vi "fp button handler_MD.vi"(5 "dummy error input (just for timing purposes)":errorcluster) -> ()   [LabVIEW 2012]
uses:
  <vilib>/Utility/VariantDataType/Type.ctl
  GFG/GFGallGet.vi
  GFG/GFGfpRefGet.vi
  GFG/GFG library.lvlib
  <vilib>/Utility/VariantDataType/VariantType.lvlib
panel:
  out "Source VI":string
  in  "stop":bool
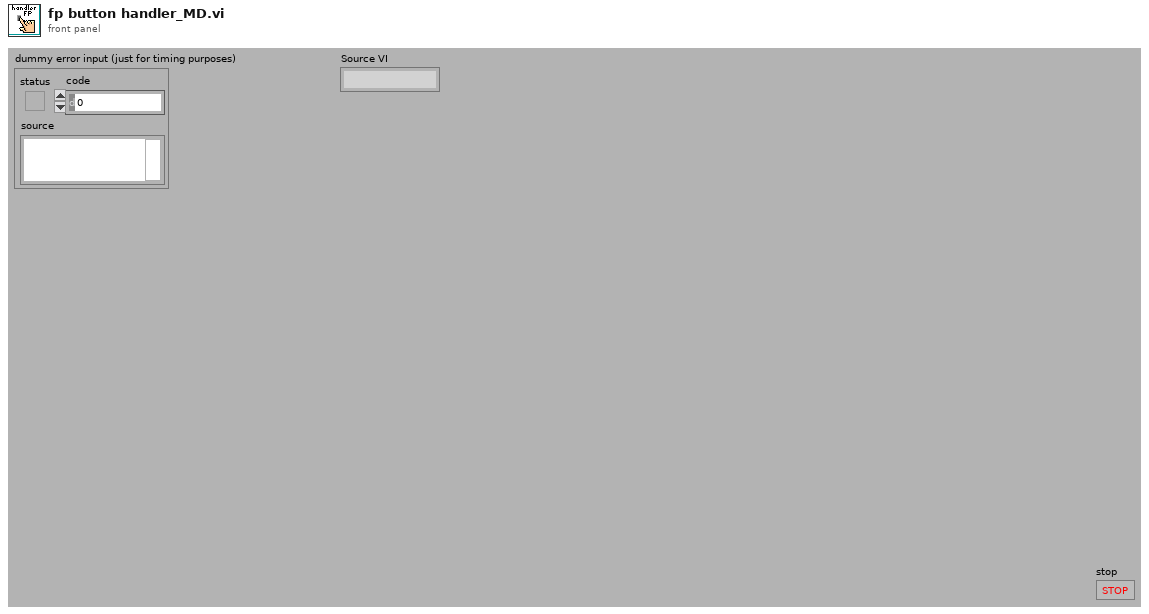
[diagram p1: front panel]
types:
  T1 = typedef "VariantType.lvlib/Type.ctl" = enum8{"Invalid Type", "Void", "I8", "I16", "I32", "I64", "U8", "U16", "U32", "U64", "Single Float", "Double Float", "Extended Float", "Single Complex", "Double Complex", "Extended Complex", "Enum U8", "Enum U16", "Enum U32", "Enum U64", "Single Float With Unit", "Double Float With Unit", "Extended Float With Unit", "Single Complex with Unit", "Double Complex with Unit", "Extended Complex with Unit", "Boolean", "String", "Path", "Picture", "Tag", "Array", "Cluster", "Variant", "LV Variant", "Waveform", "Timestamp", "Digital Waveform", "Digital Data", "ExpressData", "Refnum", "External Data", "VI", "Poly VI", "LabVIEW Class Instance", "Fixed Point"}
  T2 = cluster{"Variable Name Out":string, "Data Type Out":T1, "Variant Out":variant}[]
  T3 = cluster{"WaveformChartRef":refnum<vi>, "DigitalRef":refnum<vi>, "ArrayRef":refnum<vi>, "TabControlRef":refnum<vi>, "EnumRef":refnum<vi>, "RingRef":refnum<vi>, "BooleanRef":refnum<vi>, "KnobRef":refnum<vi>, "SlideRef":refnum<vi>, "PathRef":refnum<vi>, "StringRef":refnum<vi>, "ComboBox":refnum<vi>, "WaveformGraphRef":refnum<vi>}
  T4 = enum8{"Enabled", "Disabled", "Disabled and Grayed Out"}
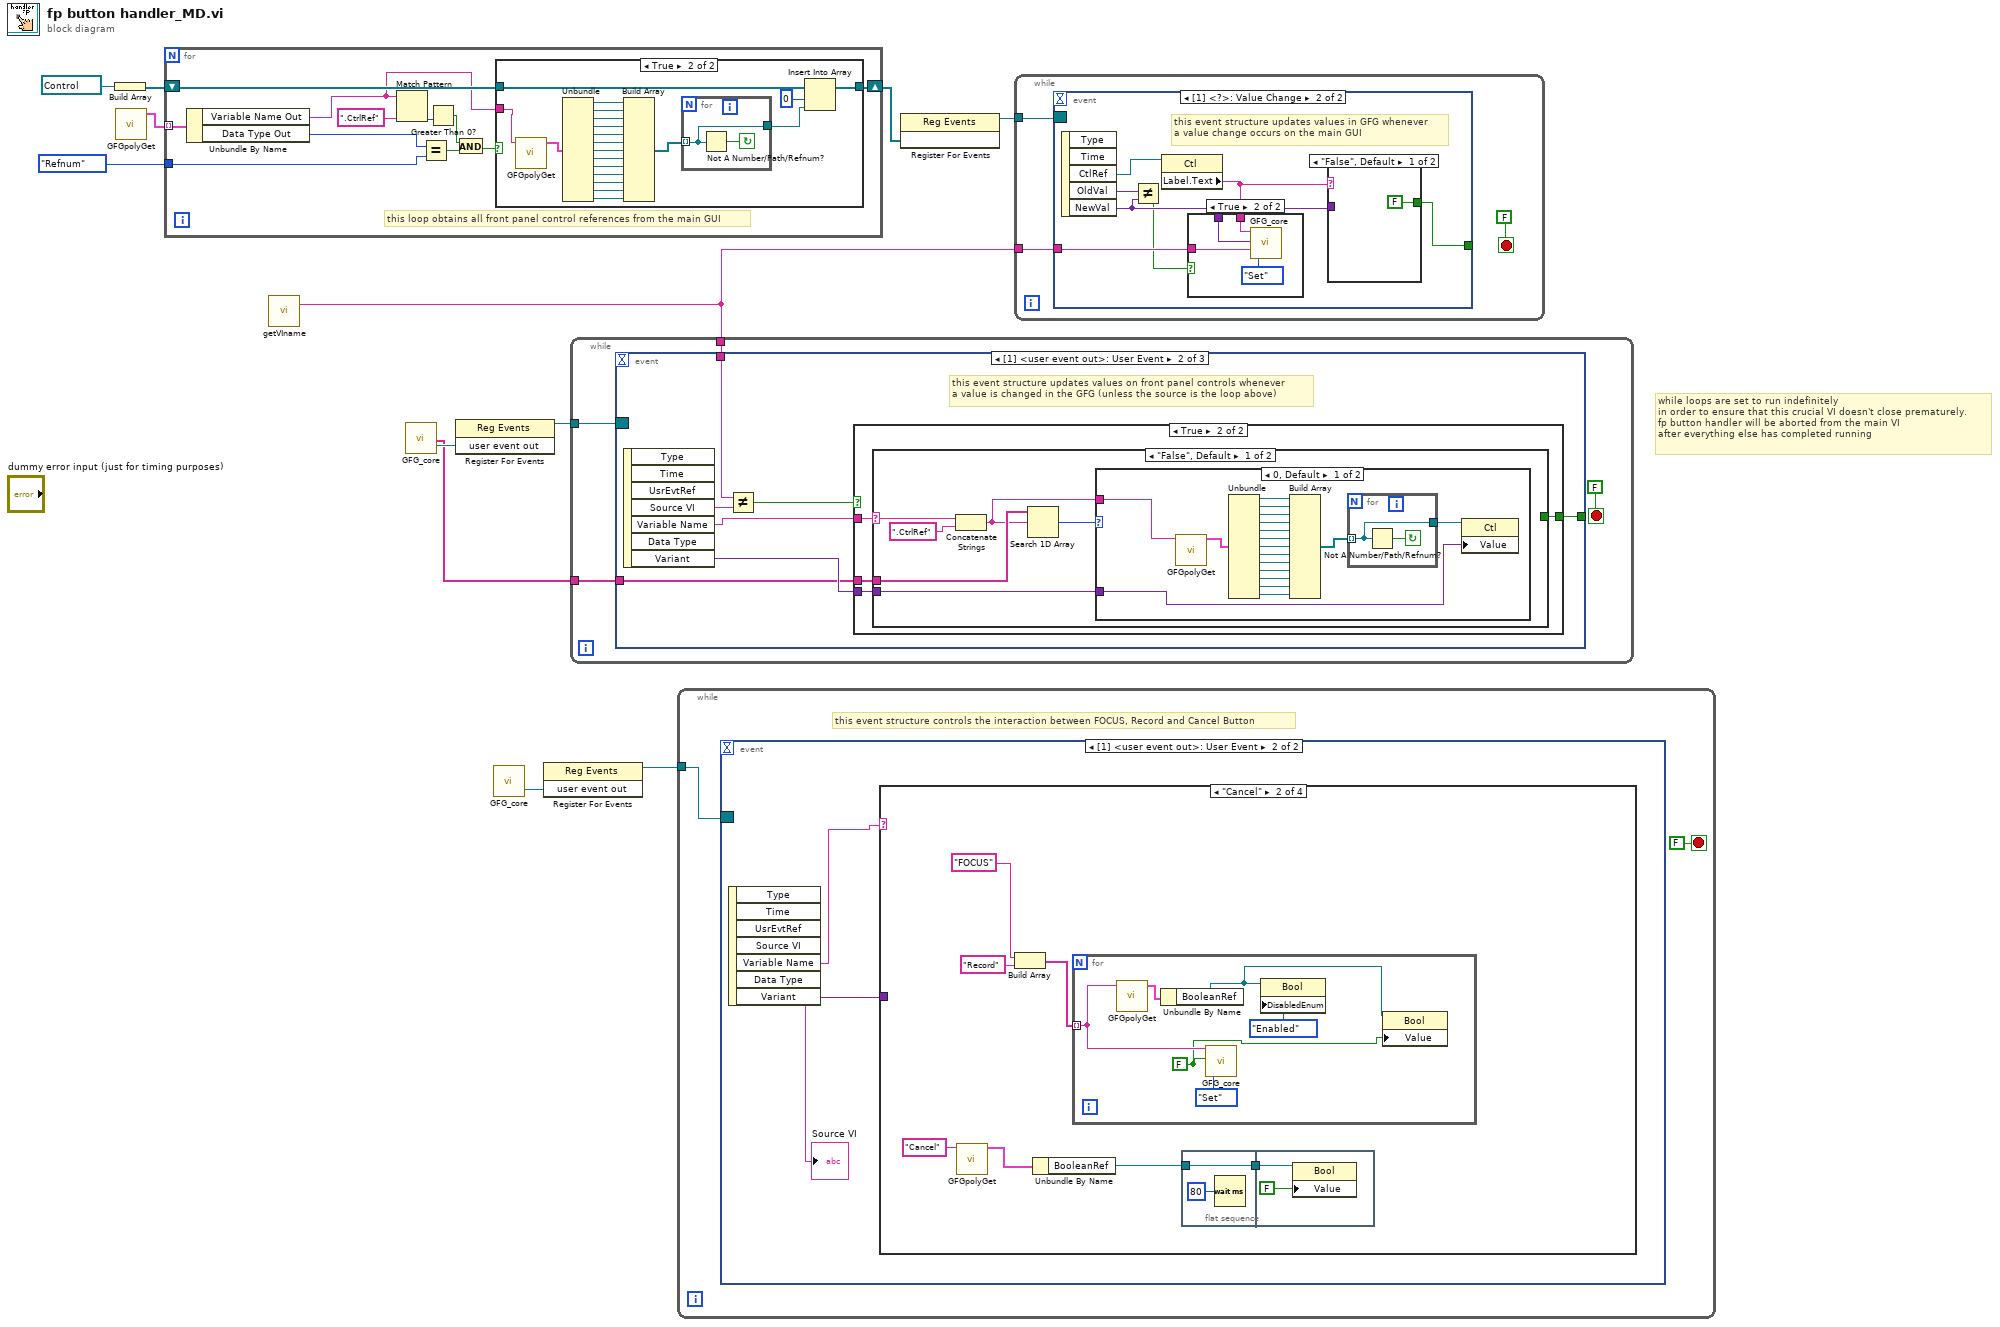
[diagram p0: block diagram]
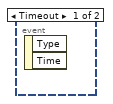
[diagram p2: hidden frame]
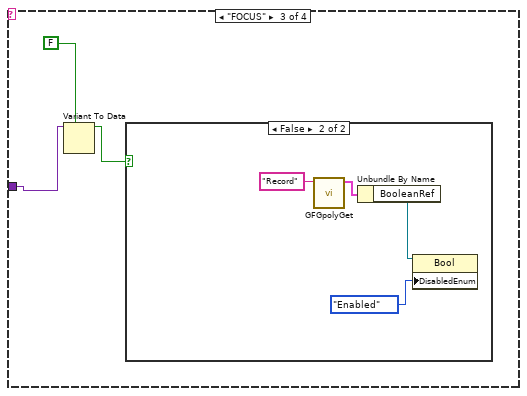
[diagram p4: hidden frame]
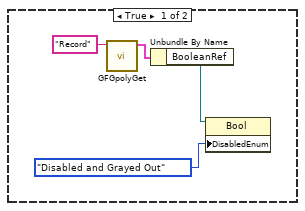
[diagram p5: hidden frame]
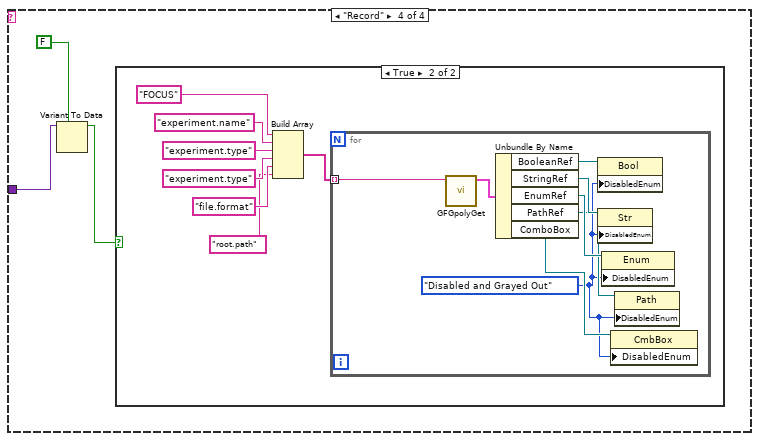
[diagram p6: hidden frame]
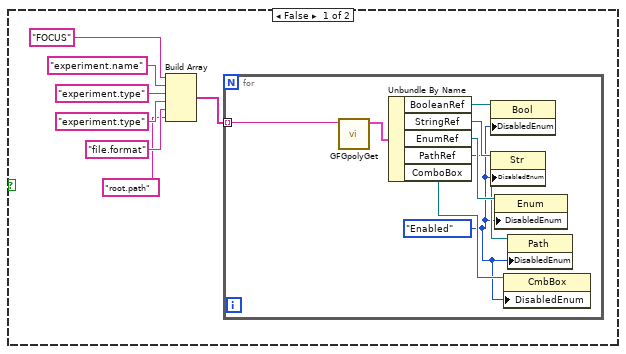
[diagram p7: hidden frame]
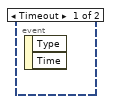
[diagram p8: hidden frame]
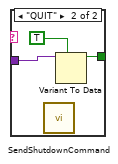
[diagram p10: hidden frame]
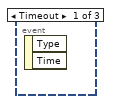
[diagram p12: hidden frame]
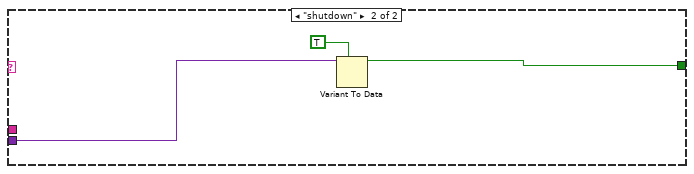
[diagram p15: hidden frame]
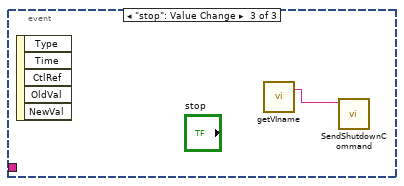
[diagram p16: hidden frame]
diagram:
  # "while loops are set to run indefinitely\nin order to ensure that this crucial VI doesn't close prematurely.\nfp button handler will be aborted from the main VI \nafter everything else has completed running"
  n1 = Build Array(refnum<vi> refnum ("DigitalRef")) -> (w6:refnum<vi>[])
  n2 = call-poly "GFGpolyGet.vi"() -> ("Array of Clusters of Variables"=w9:T2)  [unwired: 10 in, 1 out]
  n3 = for {
    tunnel: w9 -> [w23] mode=indexing
    tunnel: Type."Refnum" ("Data Type Out") -> [w21]
    shift-right: [w19] -> w5
    shift-left: w6 -> [w20]
    # "this loop obtains all front panel control references from the main GUI"
    n4 = Unbundle By Name(w23) -> ("Variable Name Out"=w13:string, "Data Type Out"=w22:T1)
    n5 = Match Pattern(string=w13, regular expression=".CtrlRef" ("string")) -> (offset past match=w17:i32)  [unwired: 1 in, 3 out]
    n6 = Equal?(x=w22, y=w21) -> (x = y?=w14:bool)
    n7 = Greater Than 0?(x=w17) -> (x > 0?=w15:bool)
    n8 = And(x=w15, y=w14) -> (x .and. y?=w16:bool)
    n9 = case shown="True" w16 {
      tunnel: w20 -> [w24 w30]
      tunnel: [w24 w29] -> w19
      tunnel: w13 -> [_ w27]
      frame False {
      }
      frame True {
        n10 = call-poly "GFGpolyGet.vi"("Variable Name in"=w27) -> ("output cluster"=w32:T3)  [unwired: 9 in, 1 out]
        n11 = Unbundle(w32) -> ("WaveformChartRef"=w33:refnum<vi>, "DigitalRef"=w34:refnum<vi>, "ArrayRef"=w35:refnum<vi>, "TabControlRef"=w36:refnum<vi>, "EnumRef"=w37:refnum<vi>, "RingRef"=w38:refnum<vi>, "BooleanRef"=w39:refnum<vi>, "KnobRef"=w40:refnum<vi>, "SlideRef"=w41:refnum<vi>, "PathRef"=w42:refnum<vi>, "StringRef"=w43:refnum<vi>, "ComboBox"=w26:refnum<vi>, "WaveformGraphRef"=w25:refnum<vi>)
        n12 = Build Array(w33, w34, w35, w36, w37, w38, w39, w40, w41, w42, w43, w26, w25) -> (w44:refnum<vi>[])
        n13 = for {
          tunnel: w44 -> [w45] mode=indexing
          tunnel: [w45] -> w31
          stop <- w46 continue-if-true
          n14 = Not A Number/Path/Refnum?(number/path/refnum=w45) -> (NaN/Path/Refnum?=w46:bool)
        }
        n15 = Insert Into Array(array=w30, index=0, new element=w31) -> (w29:refnum<vi>[])
      }
    }
  }
  n16 = call "getVIname.vi"() -> ("VI name"=w1:string)  [unwired: 19 in]
  n17 = call "GFG_core.vi"() -> ("All Variable Names Out"=w10:string[], "user event out"=w11:refnum<user-event>)  [unwired: 13 in, 5 out]
  n18 = register-events(w11) -> (reference out=w12:refnum<event-registration>)  [unwired: 2 in, 1 out]
  n19 = call "GFG_core.vi"() -> ("user event out"=w3:refnum<user-event>)  [unwired: 13 in, 6 out]
  n20 = register-events(w3) -> (reference out=w2:refnum<event-registration>)  [unwired: 2 in, 1 out]
  n21 = while {
    tunnel: w12 -> [w50]
    tunnel: w10 -> [w49]
    tunnel: w1 -> [w48]
    stop <- FALSE stop-if-true
    n22 = event shown="[1] <user event out>: User Event" {
      selector: w50 -> [_ _ _]
      dyn-events: _ -> [_ _ _]
      timeout: _ -> [_ _ _]
      tunnel: [_ w55 _] -> _
      tunnel: w49 -> [_ w54 _]
      tunnel: w48 -> [_ w53 _]
      event Timeout {
        n23 = event-data() -> ()  [unwired: 1 in, 2 out]
      }
      event User Event {
        # "this event structure updates values on front panel controls whenever\na value is changed in the GFG (unless the source is the loop above)"
        n24 = event-data() -> ("Source VI"=w52:string, "Variable Name"=w57:string, "Variant"=w56:variant)  [unwired: 1 in, 4 out]
        n25 = Not Equal?(x=w53, y=w52) -> (x != y?=w51:bool)
        n26 = case shown="True" w51 {
          tunnel: w57 -> [_ w61]
          tunnel: w56 -> [_ w60]
          tunnel: [_ w59] -> w55
          tunnel: w54 -> [_ w58]
          frame False {
          }
          frame True {
            n27 = case shown="\"False\", Default" w61 {
              selector: w61 -> [w66 _]
              tunnel: w60 -> [w62 w90]
              tunnel: [_ w88] -> w59
              tunnel: w58 -> [w65 _]
              frame "False", Default {
                n28 = Concatenate Strings(w66, ".CtrlRef" ("string")) -> (w63:string)
                n29 = Search 1D Array(1D array=w65, element=w63) -> (index of element=w64:i32)  [unwired: 1 in]
                n30 = case shown="0, Default" w64 {
                  tunnel: w63 -> [w85 _]
                  tunnel: w62 -> [w70 _]
                  frame 0, Default {
                    n31 = call-poly "GFGpolyGet.vi"("Variable Name in"=w85) -> ("output cluster"=w84:T3)  [unwired: 9 in, 1 out]
                    n32 = Unbundle(w84) -> ("WaveformChartRef"=w83:refnum<vi>, "DigitalRef"=w82:refnum<vi>, "ArrayRef"=w81:refnum<vi>, "TabControlRef"=w80:refnum<vi>, "EnumRef"=w79:refnum<vi>, "RingRef"=w78:refnum<vi>, "BooleanRef"=w77:refnum<vi>, "KnobRef"=w76:refnum<vi>, "SlideRef"=w75:refnum<vi>, "PathRef"=w74:refnum<vi>, "StringRef"=w73:refnum<vi>, "ComboBox"=w69:refnum<vi>, "WaveformGraphRef"=w68:refnum<vi>)
                    n33 = Build Array(w83, w82, w81, w80, w79, w78, w77, w76, w75, w74, w73, w69, w68) -> (w72:refnum<vi>[])
                    n34 = for {
                      tunnel: w72 -> [w86] mode=indexing
                      tunnel: [w86] -> w71
                      stop <- w87 continue-if-true
                      n35 = Not A Number/Path/Refnum?(number/path/refnum=w86) -> (NaN/Path/Refnum?=w87:bool)
                    }
                    n36 = property class="Ctl"(reference=w71, "Value"=w70) -> ()  [unwired: 1 in, 2 out]
                  }
                  frame -1 {
                  }
                }
              }
              frame "shutdown" {
                n37 = Variant To Data(type=TRUE ("want seconds? (F)"), Variant=w90) -> (data=w88:bool)  [unwired: 1 in, 1 out]
              }
            }
          }
        }
      }
      event "stop": Value Change {
        n38 = event-data() -> ()  [unwired: 1 in, 5 out]
        n39 = call "getVIname.vi"() -> ("VI name"=w91:string)  [unwired: 19 in]
        n40 = call "SendShutdownCommand.vi"("Source VI"=w91) -> ()  [unwired: 11 in]
      }
    }
  }
  n41 = while {
    tunnel: w2 -> [w93]
    stop <- FALSE stop-if-true
    # "this event structure controls the interaction between FOCUS, Record and Cancel Button"
    n42 = event shown="[1] <user event out>: User Event" {
      selector: w93 -> [_ _]
      dyn-events: _ -> [_ _]
      timeout: _ -> [_ _]
      event Timeout {
        n43 = event-data() -> ()  [unwired: 1 in, 2 out]
      }
      event User Event {
        n44 = event-data() -> ("Source VI"=→"Source VI":string, "Variable Name"=w96:string, "Variant"=w95:variant)  [unwired: 1 in, 4 out]
        n45 = case shown="\"Cancel\"" w96 {
          tunnel: w95 -> [_ _ w115 w127]
          frame "False", Default {
          }
          frame "Cancel" {
            n46 = call-poly "GFGpolyGet.vi"("Variable Name in"="Cancel") -> ("output cluster"=w99:T3)  [unwired: 9 in, 1 out]
            n47 = Build Array("FOCUS" ("Variable Name in"), "Record" ("element")) -> (w101:string[])
            n48 = Unbundle By Name(w99) -> ("BooleanRef"=w98:refnum<vi>)
            n49 = for {
              tunnel: w101 -> [w110] mode=indexing
              w108 = FALSE
              n50 = call-poly "GFGpolyGet.vi"("Variable Name in"=w110) -> ("output cluster"=w112:T3)  [unwired: 9 in, 1 out]
              n51 = Unbundle By Name(w112) -> ("BooleanRef"=w109:refnum<vi>)
              n52 = call "GFG_core.vi"("Variable Name in"=w110, "Variant in"=w108, "Action"=enum16{"Init", "Set", "Get"}."Set") -> ()  [unwired: 10 in, 7 out]
              n53 = property class="Bool"(reference=w109, "DisabledEnum"=T4."Enabled" ("Disabled")) -> ()  [unwired: 1 in, 2 out]
              n54 = property class="Bool"(reference=w109, "Value"=w108) -> ()  [unwired: 1 in, 2 out]
            }
            n55 = flat-sequence {
              tunnel: w98 -> [w105]
              tunnel: [w105] -> w97
              tunnel: w97 -> [w107]
              frame #0 {
                n56 = Wait (ms)(milliseconds to wait=u32 80) -> ()  [unwired: 1 out]
              }
              frame #1 {
                n57 = property class="Bool"(reference=w107, "Value"=FALSE) -> ()  [unwired: 1 in, 2 out]
              }
            }
          }
          frame "FOCUS" {
            n58 = Variant To Data(type=FALSE ("NewVal"), Variant=w115) -> (data=w114:bool)  [unwired: 1 in, 1 out]
            n59 = case shown="False" w114 {
              frame True {
                n60 = call-poly "GFGpolyGet.vi"("Variable Name in"="Record") -> ("output cluster"=w118:T3)  [unwired: 9 in, 1 out]
                n61 = Unbundle By Name(w118) -> ("BooleanRef"=w117:refnum<vi>)
                n62 = property class="Bool"(reference=w117, "DisabledEnum"=T4."Disabled and Grayed Out" ("Disabled")) -> ()  [unwired: 1 in, 2 out]
              }
              frame False {
                n63 = call-poly "GFGpolyGet.vi"("Variable Name in"="Record") -> ("output cluster"=w122:T3)  [unwired: 9 in, 1 out]
                n64 = Unbundle By Name(w122) -> ("BooleanRef"=w121:refnum<vi>)
                n65 = property class="Bool"(reference=w121, "DisabledEnum"=T4."Enabled" ("Disabled")) -> ()  [unwired: 1 in, 2 out]
              }
            }
          }
          frame "Record" {
            n66 = Variant To Data(type=FALSE ("NewVal"), Variant=w127) -> (data=w125:bool)  [unwired: 1 in, 1 out]
            n67 = case shown="True" w125 {
              frame False {
                n68 = Build Array("FOCUS" ("Variable Name in"), "experiment.name" ("element"), "experiment.type" ("element"), "experiment.type" ("element"), "file.format" ("element"), "root.path" ("element")) -> (w129:string[])
                n69 = for {
                  tunnel: w129 -> [w140] mode=indexing
                  w135 = T4."Enabled" ("Disabled")
                  n70 = call-poly "GFGpolyGet.vi"("Variable Name in"=w140) -> ("output cluster"=w142:T3)  [unwired: 9 in, 1 out]
                  n71 = Unbundle By Name(w142) -> ("BooleanRef"=w141:refnum<vi>, "StringRef"=w139:refnum<vi>, "EnumRef"=w138:refnum<vi>, "PathRef"=w137:refnum<vi>, "ComboBox"=w136:refnum<vi>)
                  n72 = property class="Bool"(reference=w141, "DisabledEnum"=w135) -> ()  [unwired: 1 in, 2 out]
                  n73 = property class="Str"(reference=w139, "DisabledEnum"=w135) -> ()  [unwired: 1 in, 2 out]
                  n74 = property class="Enum"(reference=w138, "DisabledEnum"=w135) -> ()  [unwired: 1 in, 2 out]
                  n75 = property class="CmbBox"(reference=w136, "DisabledEnum"=w135) -> ()  [unwired: 1 in, 2 out]
                  n76 = property class="Path"(reference=w137, "DisabledEnum"=w135) -> ()  [unwired: 1 in, 2 out]
                }
              }
              frame True {
                n77 = Build Array("FOCUS" ("Variable Name in"), "experiment.name" ("element"), "experiment.type" ("element"), "experiment.type" ("element"), "file.format" ("element"), "root.path" ("element")) -> (w144:string[])
                n78 = for {
                  tunnel: w144 -> [w155] mode=indexing
                  w150 = T4."Disabled and Grayed Out" ("Disabled")
                  n79 = call-poly "GFGpolyGet.vi"("Variable Name in"=w155) -> ("output cluster"=w157:T3)  [unwired: 9 in, 1 out]
                  n80 = Unbundle By Name(w157) -> ("BooleanRef"=w156:refnum<vi>, "StringRef"=w154:refnum<vi>, "EnumRef"=w153:refnum<vi>, "PathRef"=w152:refnum<vi>, "ComboBox"=w151:refnum<vi>)
                  n81 = property class="Bool"(reference=w156, "DisabledEnum"=w150) -> ()  [unwired: 1 in, 2 out]
                  n82 = property class="Str"(reference=w154, "DisabledEnum"=w150) -> ()  [unwired: 1 in, 2 out]
                  n83 = property class="Enum"(reference=w153, "DisabledEnum"=w150) -> ()  [unwired: 1 in, 2 out]
                  n84 = property class="CmbBox"(reference=w151, "DisabledEnum"=w150) -> ()  [unwired: 1 in, 2 out]
                  n85 = property class="Path"(reference=w152, "DisabledEnum"=w150) -> ()  [unwired: 1 in, 2 out]
                }
              }
            }
          }
        }
      }
    }
  }
  n86 = register-events(w5) -> (reference out=w4:refnum<event-registration>)  [unwired: 2 in, 1 out]
  n87 = while {
    tunnel: w4 -> [w160]
    tunnel: w1 -> [w159]
    stop <- FALSE stop-if-true
    n88 = event shown="[1] <?>: Value Change" {
      selector: w160 -> [_ _]
      dyn-events: _ -> [_ _]
      timeout: _ -> [_ _]
      tunnel: w159 -> [_ w166]
      tunnel: [_ w164] -> _
      event Timeout {
        n89 = event-data() -> ()  [unwired: 1 in, 2 out]
      }
      event Value Change {
        # "this event structure updates values in GFG whenever\na value change occurs on the main GUI"
        n90 = event-data() -> ("CtlRef"=w167:refnum<vi>, "OldVal"=w163:variant, "NewVal"=w162:variant)  [unwired: 1 in, 2 out]
        n91 = Not Equal?(x=w163, y=w162) -> (x != y?=w161:bool)
        n92 = property class="Ctl"(reference=w167) -> ("Label.Text"=w165:string)  [unwired: 1 in, 2 out]
        n93 = case shown="True" w161 {
          tunnel: w166 -> [_ w170]
          tunnel: w165 -> [_ w169]
          tunnel: w162 -> [_ w168]
          frame False {
          }
          frame True {
            n94 = call "GFG_core.vi"("Variable Name in"=w169, "Variant in"=w168, "Source VI"=w170, "Action"=enum16{"Init", "Set", "Get"}."Set") -> ()  [unwired: 9 in, 7 out]
          }
        }
        n95 = case shown="\"False\", Default" w165 {
          tunnel: w162 -> [_ w175]
          tunnel: [FALSE w173] -> w164
          frame "False", Default {
          }
          frame "QUIT" {
            n96 = call "SendShutdownCommand.vi"() -> ()  [unwired: 12 in]
            n97 = Variant To Data(type=TRUE, Variant=w175) -> (data=w173:bool)  [unwired: 1 in, 1 out]
          }
        }
      }
    }
  }
